vi "未命名 1.vi"() -> ()   [LabVIEW 2017]
uses:
  <vilib>/Utility/miscctls.llb/LVBoundsTypeDef.ctl
panel:
  in  "选项卡控件":enum32{"选项卡 1", "werwer"}(tab)
  in  "树形":string(tree)
  in  "菜单下拉列表":u16(ring)
  in  "下拉列表":u16(ring)
  in  "独立标签":bool
  out "说明信息":string
  out "提示框":string
  out "选项卡标签":string
  out "选项卡标题":string
  out "选项卡可见":bool
  in  "选项卡名称":string[](array[string])
  in  "分隔栏位置":i32
  in  "容器边界":T1
  in  "颜色盒":u32(colorbox)=12189440
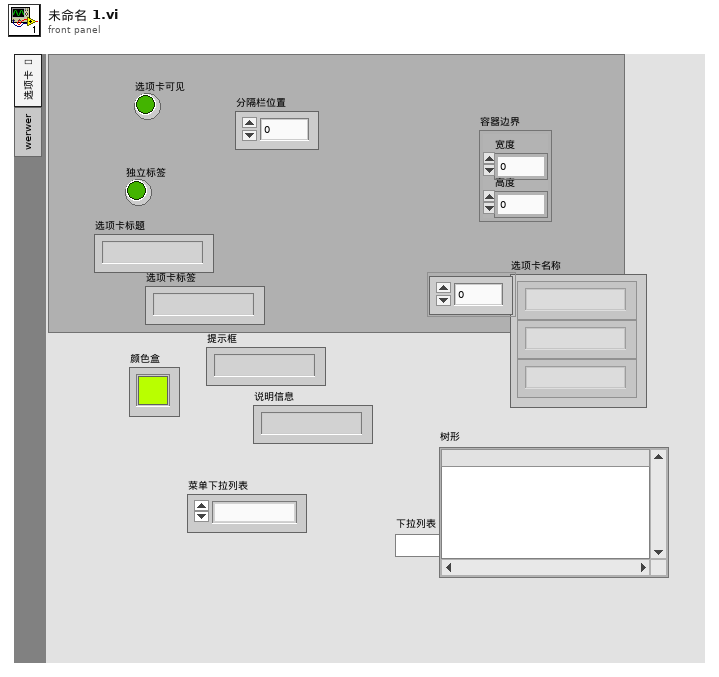
[diagram p1: front panel]
types:
  T1 = typedef "LVBoundsTypeDef.ctl" = cluster{"Width":u32, "Height":u32}
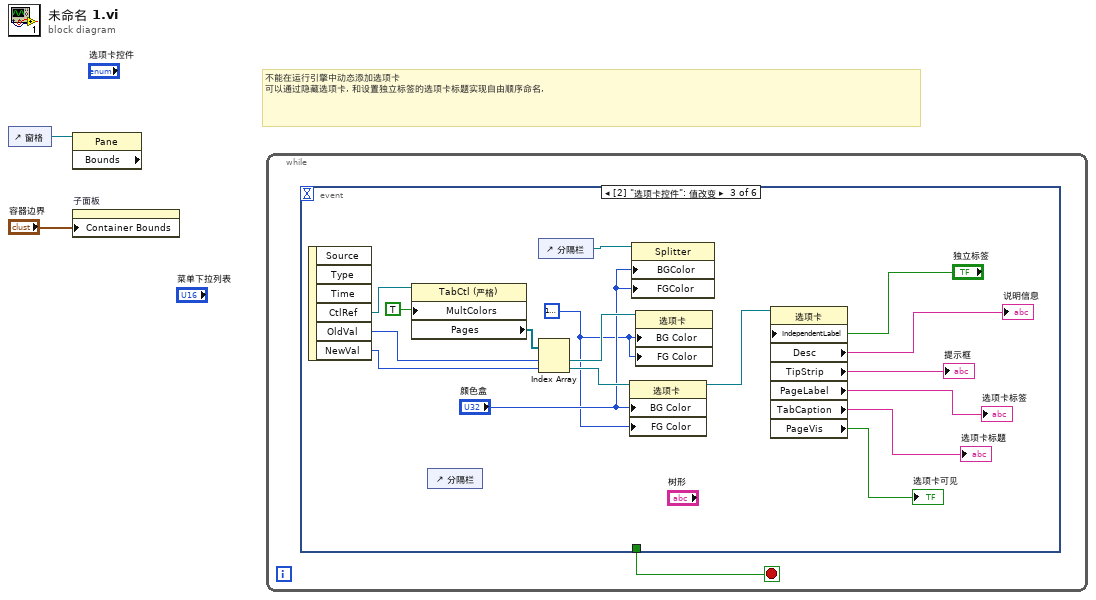
[diagram p0: block diagram]
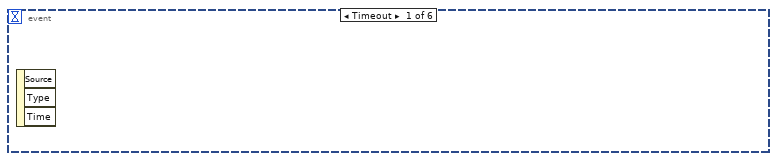
[diagram p2: hidden frame]
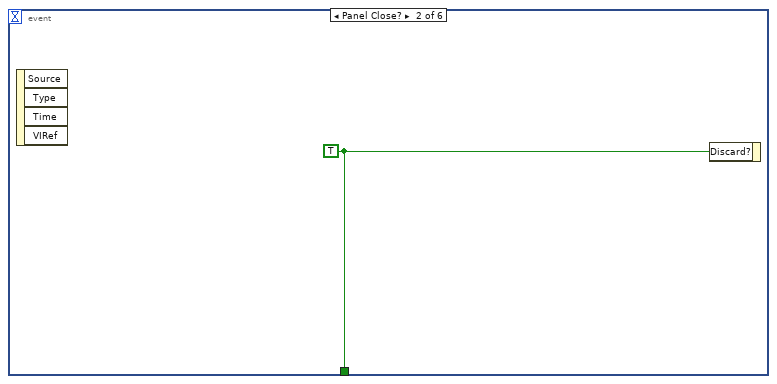
[diagram p3: hidden frame]
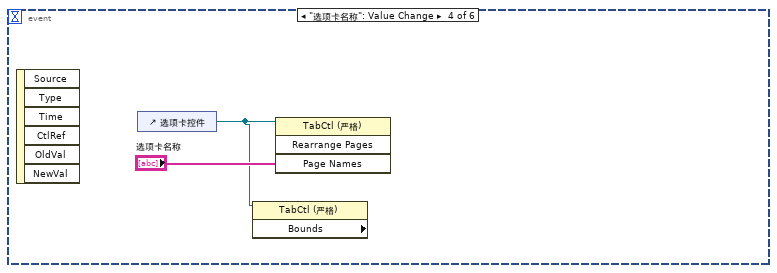
[diagram p4: hidden frame]
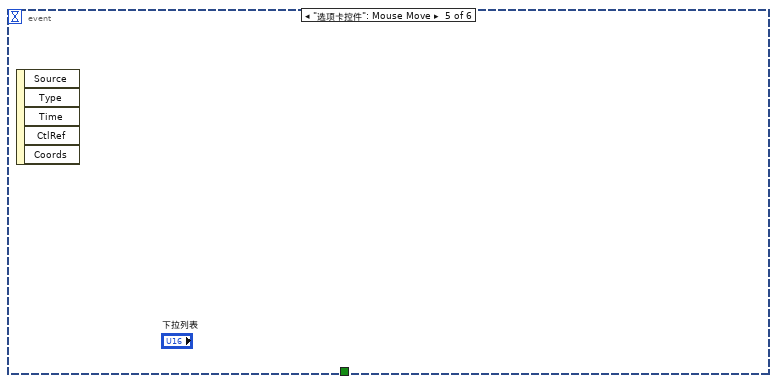
[diagram p5: hidden frame]
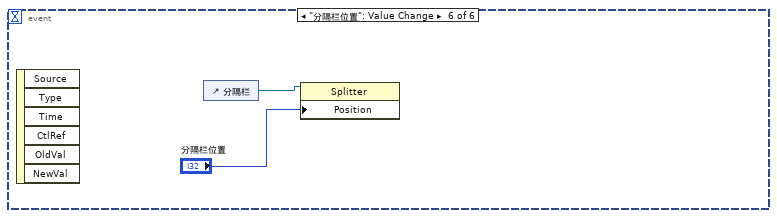
[diagram p6: hidden frame]
diagram:
  # "不能在运行引擎中动态添加选项卡\n可以通过隐藏选项卡, 和设置独立标签的选项卡标题实现自由顺序命名,"
  n1 = control-ref of="窗格"() -> (w2:refnum<vi>)
  n2 = property on="属性节点" class="Pane" props=["Bounds"](reference=w2) -> ()  [unwired: 1 in, 3 out]
  n3 = property on="子面板" class="SubPnl"("Container Bounds"="容器边界") -> ()  [unwired: 2 in, 2 out]
  n4 = while {
    stop <- w3 stop-if-true
    n5 = event shown="[2] \"选项卡控件\": 值改变" {
      selector: _ -> [_ _ _ _ _ _]
      dyn-events: _ -> [_ _ _ _ _ _]
      timeout: _ -> [_ _ _ _ _ _]
      tunnel: [_ w4 _ _ _ _] -> w3
      event Timeout {
        n6 = event-data() -> ()  [unwired: 1 in, 3 out]
      }
      event Panel Close? {
        w4 = TRUE ("放弃？")
        n7 = event-data() -> ()  [unwired: 1 in, 4 out]
        n8 = event-data("Discard?"=w4) -> ()  [unwired: 1 in, 1 out]
      }
      event "选项卡控件": Value Change {
        w12 = u32 16777216 ("颜色盒")
        n9 = event-data() -> ("CtlRef"=w21:refnum<vi>, "OldVal"=w16:enum32{"选项卡 1", "werwer"}, "NewVal"=w20:enum32{"选项卡 1", "werwer"})  [unwired: 1 in, 3 out]
        n10 = property on="属性节点" class="TabCtl (严格)"(reference=w21, "MultColors"=TRUE ("允许多种颜色")) -> ("Pages"=w19:refnum<vi>[])  [unwired: 1 in, 2 out]
        n11 = control-ref of="分隔栏"() -> ()  [unwired: 1 out]
        n12 = control-ref of="分隔栏"() -> (w14:refnum<vi>)
        n13 = Index Array(array=w19, index #1=w16, index #2=w20) -> (element #1=w15:refnum<vi>, element #2=w18:refnum<vi>)
        n14 = property class="选项卡"(reference=w18, "BG Color"="颜色盒", "FG Color"=w12) -> (reference out=w5:refnum<vi>)  [unwired: 1 in, 1 out]
        n15 = property class="Splitter"(reference=w14, "BGColor"="颜色盒", "FGColor"="颜色盒") -> ()  [unwired: 1 in, 2 out]
        n16 = property class="选项卡"(reference=w15, "BG Color"=w12, "FG Color"=w12) -> ()  [unwired: 1 in, 2 out]
        n17 = property class="选项卡"(reference=w5, "IndependentLabel"="独立标签") -> ("Desc"=→"说明信息":string, "TipStrip"=→"提示框":string, "PageLabel"=→"选项卡标签":string, "TabCaption"=→"选项卡标题":string, "PageVis"=→"选项卡可见":bool)  [unwired: 1 in, 2 out]
      }
      event "选项卡名称": Value Change {
        n18 = event-data() -> ()  [unwired: 1 in, 6 out]
        n19 = control-ref of="选项卡控件"() -> (w22:refnum<vi>)
        n20 = property on="属性节点" class="TabCtl (严格)" props=["Bounds"](reference=w22) -> ()  [unwired: 1 in, 3 out]
        n21 = invoke class="TabCtl (严格)" method="Rearrange Pages"(reference=w22, "Page Names"="选项卡名称") -> ()  [unwired: 2 in, 4 out]
      }
      event "选项卡控件": Mouse Move {
        n22 = event-data() -> ()  [unwired: 1 in, 5 out]
      }
      event "分隔栏位置": Value Change {
        n23 = event-data() -> ()  [unwired: 1 in, 6 out]
        n24 = control-ref of="分隔栏"() -> (w25:refnum<vi>)
        n25 = property class="Splitter"(reference=w25, "Position"="分隔栏位置") -> ()  [unwired: 1 in, 2 out]
      }
    }
  }
